vi "GDSString_SplitStrings.vi"(9 "MaxCharactersPerRow(25)":i32=25, 10 "StringIn":string) -> (2 "String Out":string)   [LabVIEW 2020]
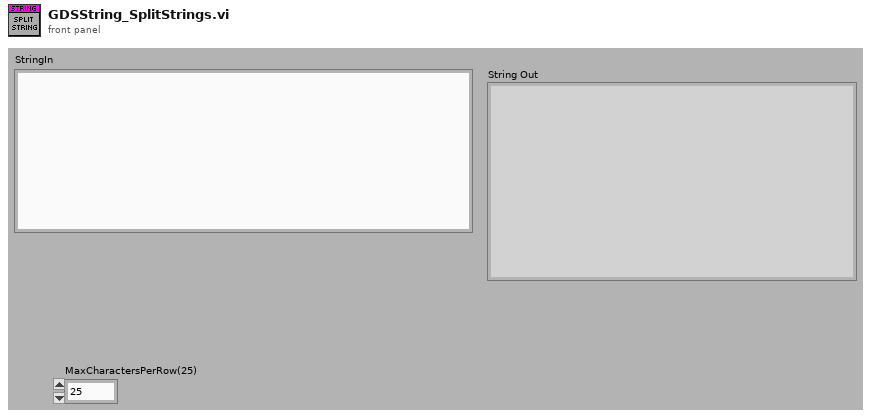
[diagram p1: front panel]
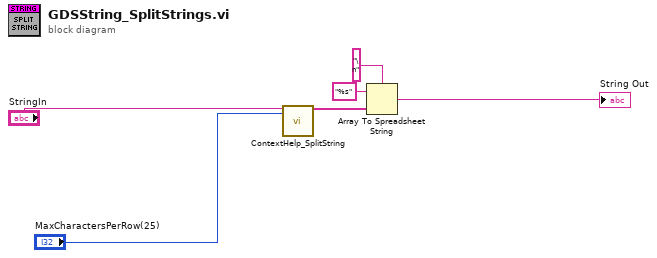
[diagram p0: block diagram]
diagram:
  n1 = call <resource>:"ContextHelp_SplitString.vi"("string"="StringIn", "Max string length"="MaxCharactersPerRow(25)") -> ("Array"=w4:string[])  [unwired: 17 in]
  n2 = Array To Spreadsheet String(delimiter (Tab)="\n", array=w4, 3:"%s" ("format string")) -> (spreadsheet string=→"String Out":string)
